vi "Catch Error.vi"(8 "Error In":errorcluster, 11 "Severity":T1) -> (0 "Error Out":errorcluster)   [LabVIEW 2014, in "Logger.lvlib"]
uses:
  Logger.lvlib
  Controls/Severity.ctl
  <vilib>/Utility/error.llb/DialogType.ctl
  Private/_Error Handler Configuration Action.ctl
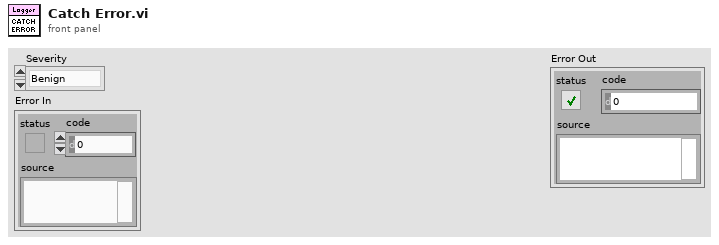
[diagram p1: front panel]
types:
  T1 = typedef "Logger.lvlib/Severity.ctl" = enum16{"Benign", "Warning", "Recoverable", "Fatal"}
  T2 = typedef "Logger.lvlib/_Error Handler Configuration Action.ctl" = enum16{"Initialize", "Get", "Set Verbosity", "Set User-Defined Codes", "Set User-Defined Descriptions", "Shutdown"}
  T3 = typedef "DialogType.ctl" = u16
  T4 = typedef "Logger.lvlib/_Error Handler Configuration.ctl" = cluster{"Verbosity":u8, "User-Defined Codes":i32[], "User-Defined Descriptions":string[]}
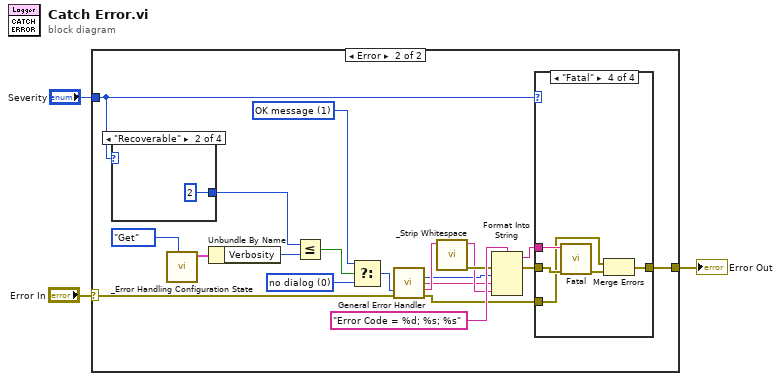
[diagram p0: block diagram]
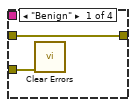
[diagram p3: hidden frame]
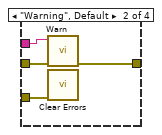
[diagram p4: hidden frame]
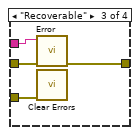
[diagram p5: hidden frame]
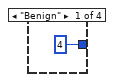
[diagram p6: hidden frame]
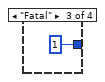
[diagram p7: hidden frame]
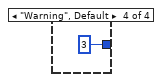
[diagram p8: hidden frame]
diagram:
  n1 = case shown="Error" "Error In" {
    selector: "Error In" -> [w4 w24]
    tunnel: "Severity" -> [_ w13]
    tunnel: [w4 w10] -> w1
    frame No Error {
    }
    frame Error {
      w23 = T3 0 items=["no dialog", "OK message", "continue or stop message", "OK message + warnings", "continue/stop + warnings"] ("type of dialog (OK msg:1)")
      w22 = T3 1 items=["no dialog", "OK message", "continue or stop message", "OK message + warnings", "continue/stop + warnings"] ("type of dialog (OK msg:1)")
      n2 = case shown="\"Recoverable\"" w13 {
        tunnel: [u8 4 u8 2 u8 1 u8 3] -> w7
        frame "Benign" {
        }
        frame "Recoverable" {
        }
        frame "Fatal" {
        }
        frame "Warning", Default {
        }
      }
      n3 = call "_Error Handling Configuration State.vi"("Action"=_Error_Handler_Configuration_Action."Get") -> ("Data"=w6:T4)  [unwired: 9 in, 1 out]
      n4 = Unbundle By Name(w6) -> ("Verbosity"=w5:u8)
      n5 = Less Or Equal?(x=w7, y=w5) -> (x <= y?=w21:bool)
      n6 = Select(t=w22, s=w21, f=w23) -> (s? t:f=w20:T3)
      n7 = call <vilib>:"General Error Handler.vi"("type of dialog (OK msg:1)"=w20, "error in (no error)"=w24) -> ("code out"=w14:i32, "source out"=w15:string, "message"=w18:string, "error out"=w12:errorcluster)  [unwired: 9 in, 1 out]
      n8 = call "_Strip Whitespace.vi"("Text"=w18) -> ("Error Out"=w17:errorcluster, "Stripped Text"=w16:string)  [unwired: 9 in]
      n9 = Format Into String(format string="Error Code = %d; %s; %s", error in=w17, w14, w15, w16) -> (resulting string=w9:string, error out=w11:errorcluster)  [unwired: 1 in]
      n10 = case shown="\"Fatal\"" w13 {
        tunnel: w12 -> [w26 w30 w31 w35]
        tunnel: w11 -> [w25 w29 w33 w39]
        tunnel: [w25 w27 w32 w36] -> w10
        tunnel: w9 -> [_ w28 w34 w38]
        frame "Benign" {
          n11 = call <vilib>:"Clear Errors.vi"("error in (no error)"=w26) -> ()  [unwired: 5 in, 2 out]
        }
        frame "Warning", Default {
          n12 = call "Warn.vi"("Error In"=w29, "Text"=w28) -> ("Error Out"=w27:errorcluster)  [unwired: 9 in]
          n13 = call <vilib>:"Clear Errors.vi"("error in (no error)"=w30) -> ()  [unwired: 5 in, 2 out]
        }
        frame "Recoverable" {
          n14 = call "Error.vi"("Error In"=w33, "Text"=w34) -> ("Error Out"=w32:errorcluster)  [unwired: 9 in]
          n15 = call <vilib>:"Clear Errors.vi"("error in (no error)"=w31) -> ()  [unwired: 5 in, 2 out]
        }
        frame "Fatal" {
          n16 = call "Fatal.vi"("Error In"=w39, "Text"=w38) -> ("Error Out"=w37:errorcluster)  [unwired: 9 in]
          n17 = Merge Errors(w35, w37) -> (w36:errorcluster)
        }
      }
    }
  }
  "Error Out" <- w1
